vi "measure stable current.vi"(6 "measure transmission?":bool, 7 "na/V 2":dbl=1000.0, 8 "error in":errorcluster, 9 "measure ss":bool, 10 "field change wait(s)":u32=5, 11 "na/V":dbl=500.0) -> (0 "error out":errorcluster, 1 "stable current 2":dbl format="%.2f", 3 "stable current":dbl format="%.2f", 4 "inj current":dbl format="%#_6e", 5 "INJ ss ratio":dbl format="%#_6e")   [LabVIEW 2016]
uses:
  stable controls/stable cluster.ctl
  kubley/data acquisition 2009/beamline/controls/stable state combo.ctl
panel:
  in  "Start.Delay":dbl=2.0 format="%#_13g"
  in  "Charge State":dbl=3.0
  out "Waveform Graph 2":dbl[](graph)
  in  "stable data in":T1={"injector current"=1.0, "offset current"=1.0, "ss inj ratio"=1.0, "ss offset ratio"=1.0, "transmission"=1.0, "2nd offset current"=1.0}
  out "stable data out":T1={"injector current"=1.0, "offset current"=1.0, "ss inj ratio"=1.0, "ss offset ratio"=1.0, "transmission"=1.0, "2nd offset current"=1.0}
  out "stable current 3":cluster{"data":dbl[]}[](graph)
  in  "inj current 4":dbl
  out "inj current 3":dbl format="%#_6e"
  in  "inj current 2":dbl
  out "step":string
  in  "measure stable":bool
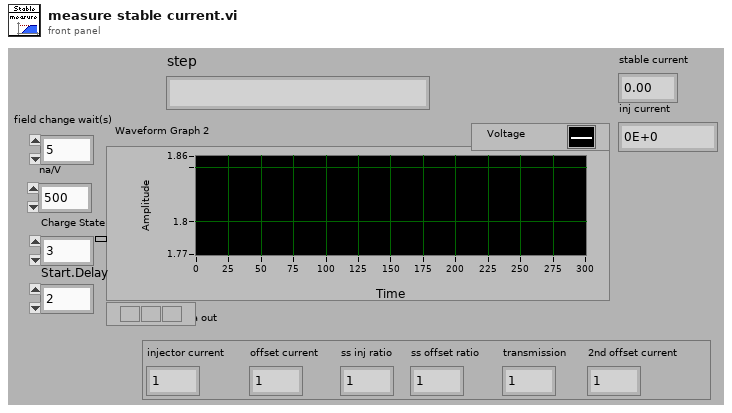
[diagram p1: front panel]
types:
  T1 = typedef "stable cluster.ctl" = cluster{"injector current":dbl, "offset current":dbl, "ss inj ratio":dbl, "ss offset ratio":dbl, "transmission":dbl, "2nd offset current":dbl}
  T2 = typedef "stable state combo.ctl" = string
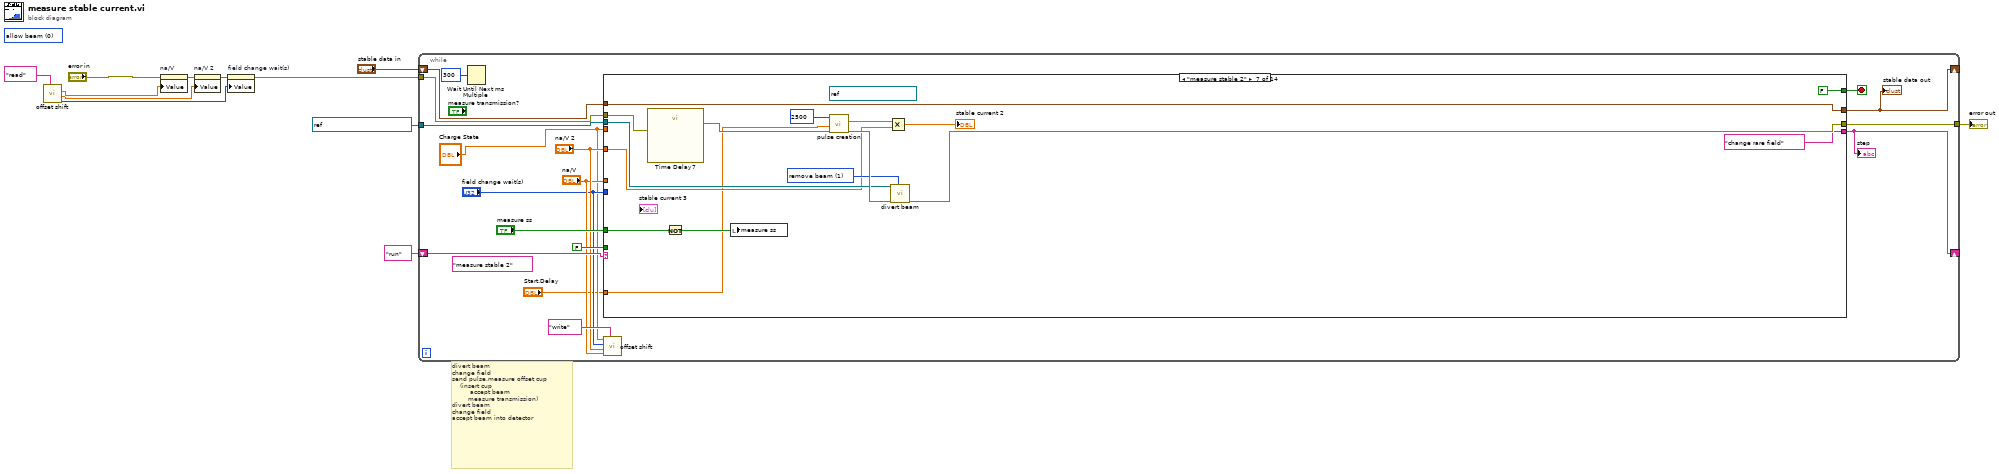
[diagram p0: block diagram]
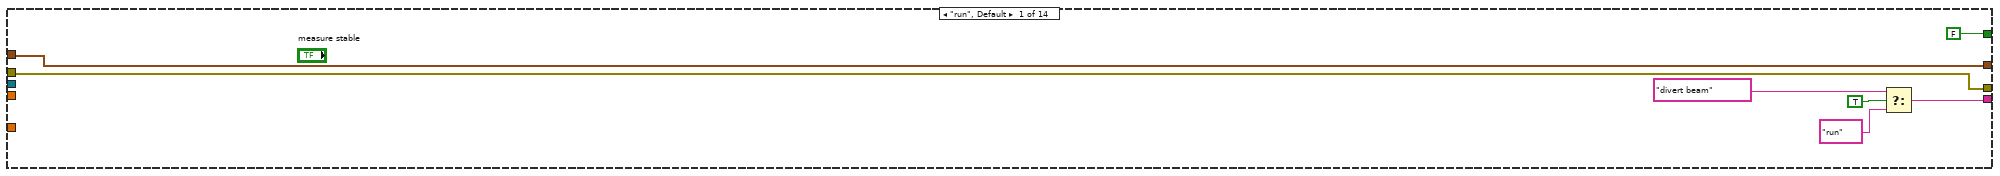
[diagram p2: hidden frame]
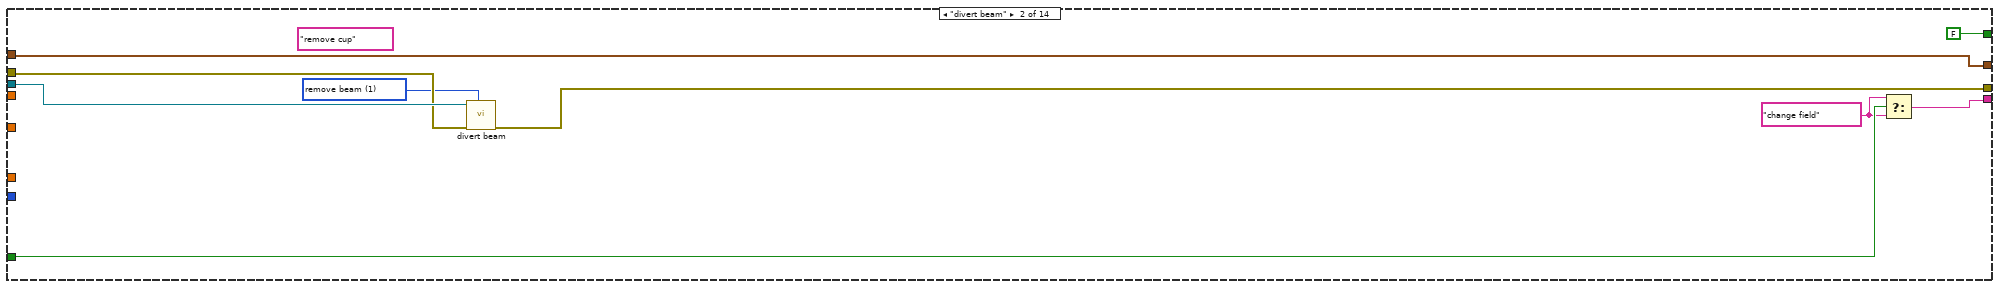
[diagram p3: hidden frame]
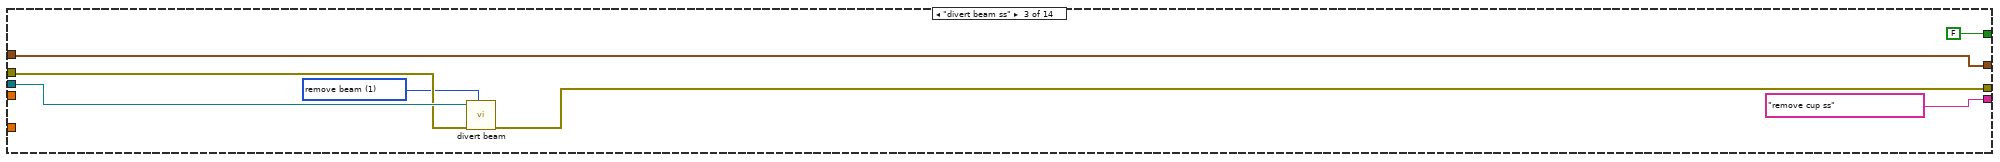
[diagram p4: hidden frame]
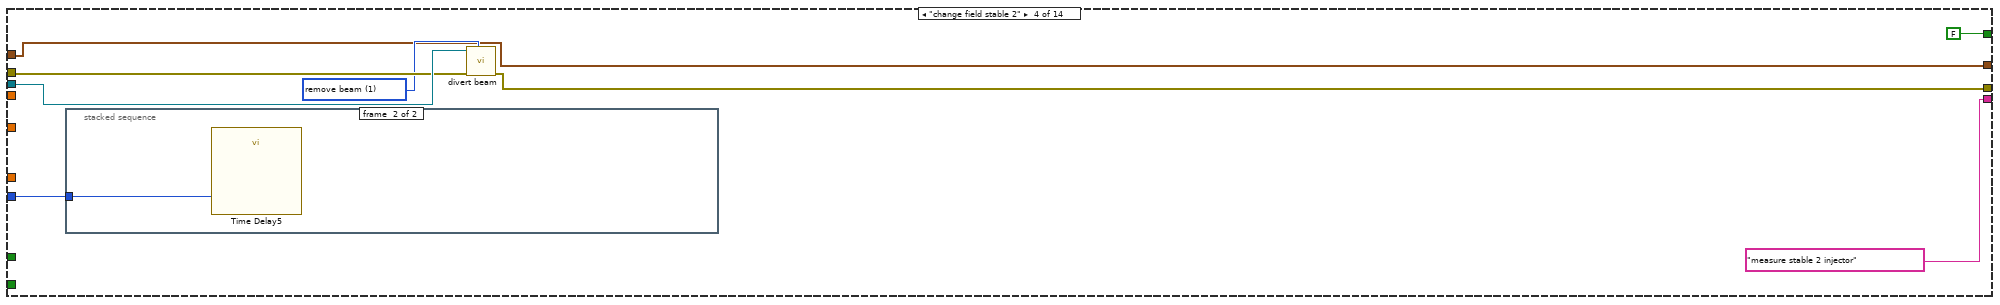
[diagram p5: hidden frame]
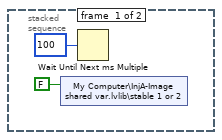
[diagram p6: hidden frame]
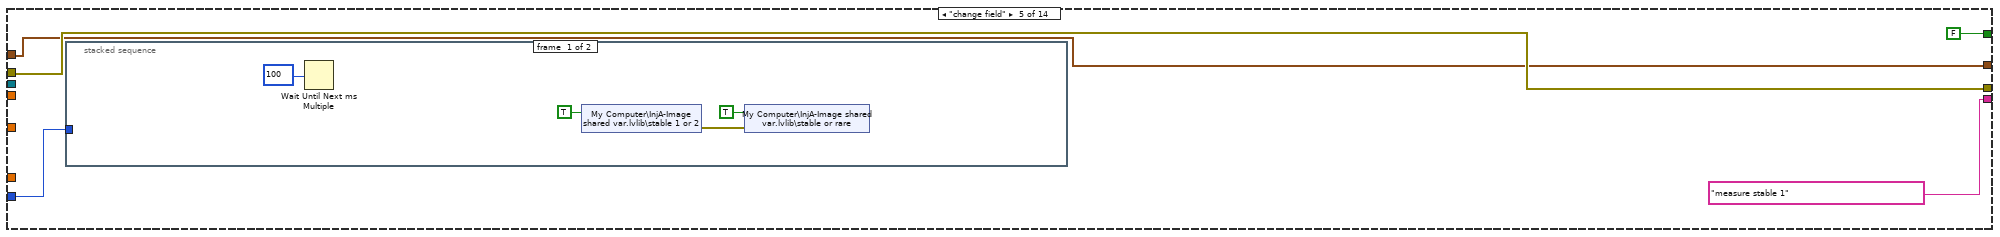
[diagram p7: hidden frame]
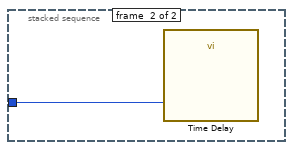
[diagram p8: hidden frame]
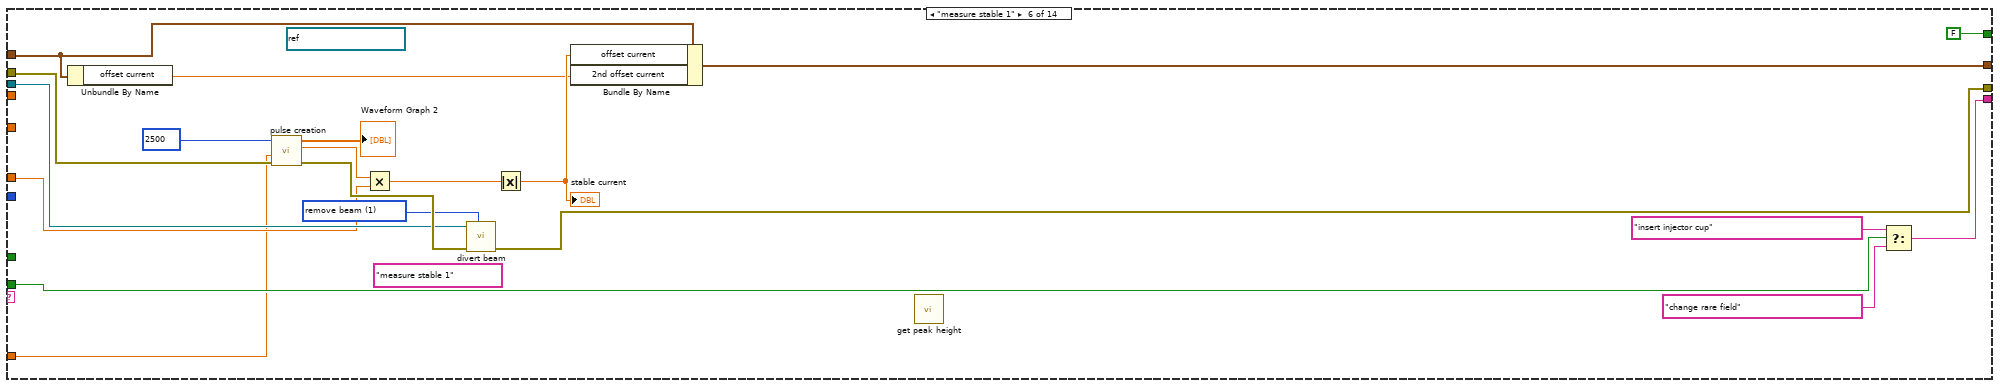
[diagram p9: hidden frame]
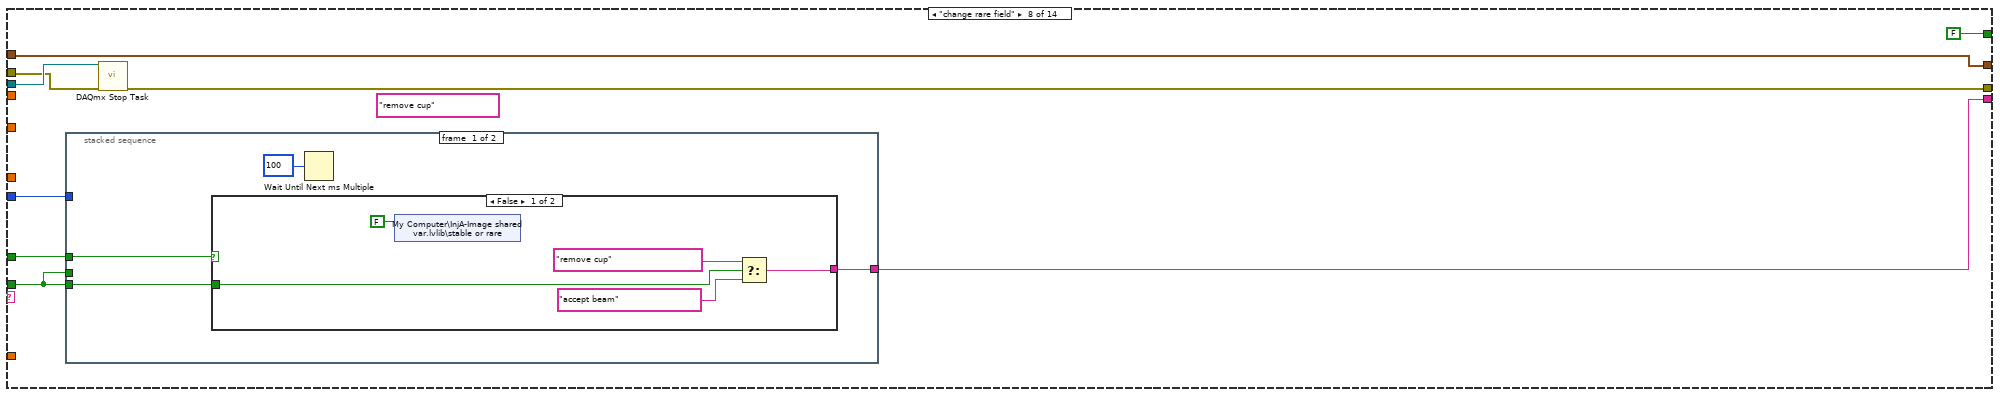
[diagram p10: hidden frame]
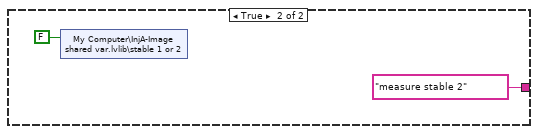
[diagram p11: hidden frame]
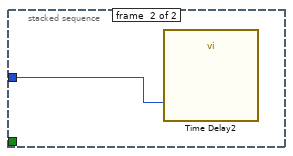
[diagram p12: hidden frame]
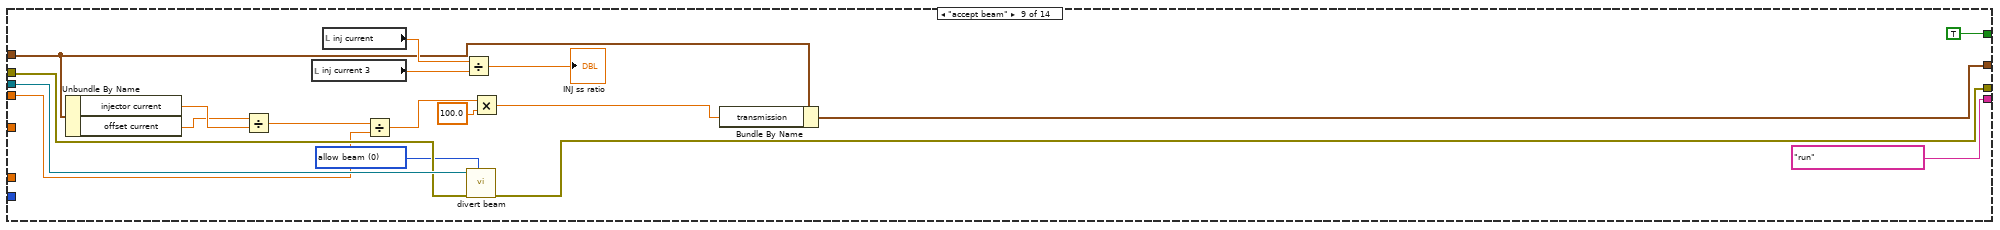
[diagram p13: hidden frame]
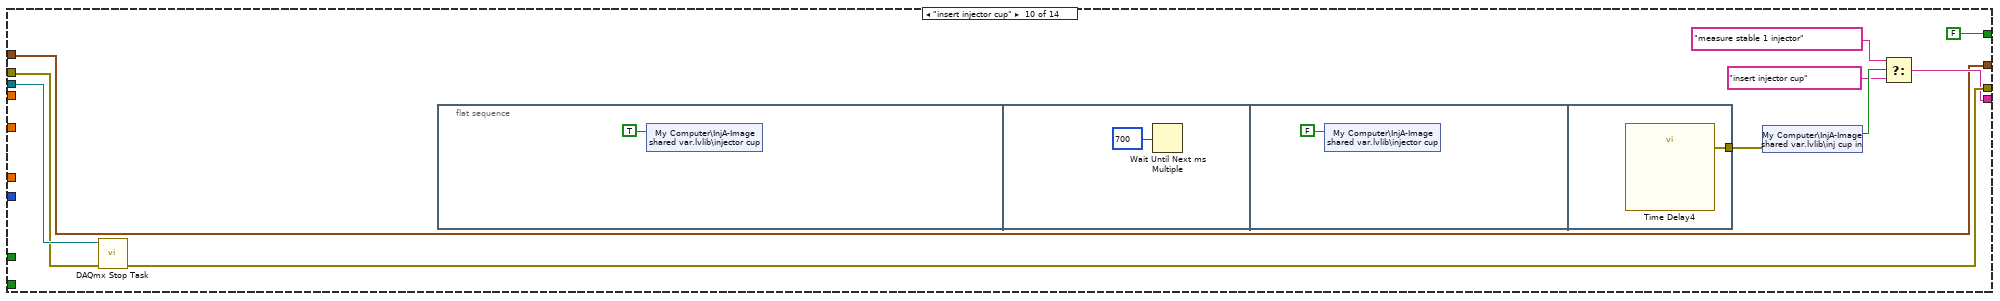
[diagram p14: hidden frame]
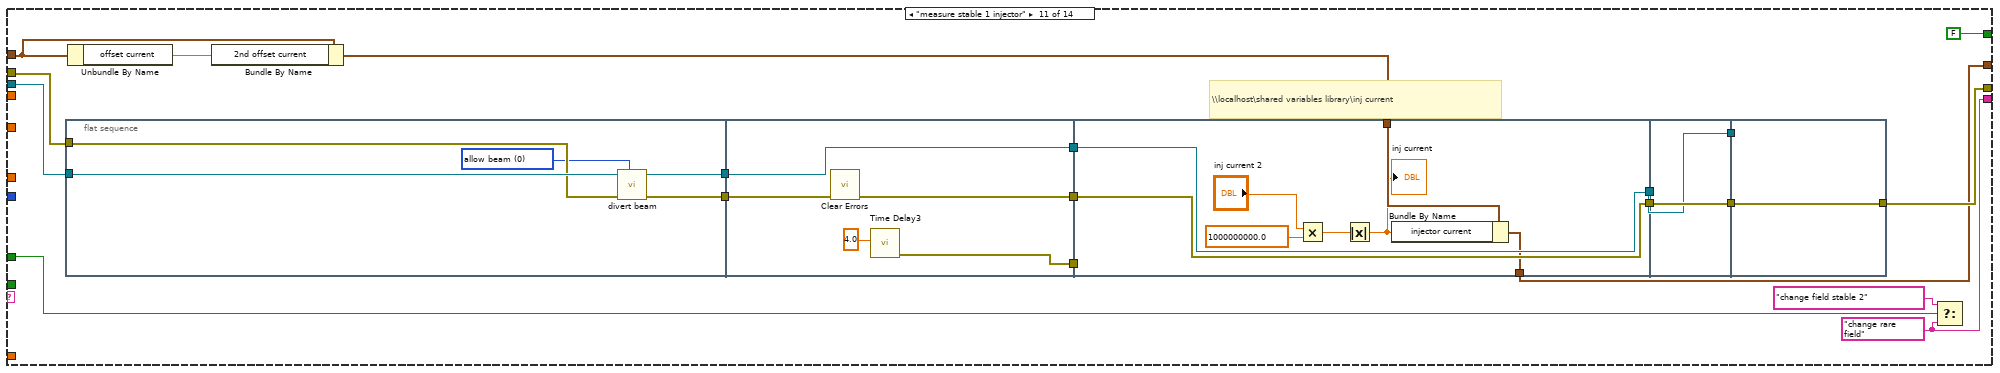
[diagram p15: hidden frame]
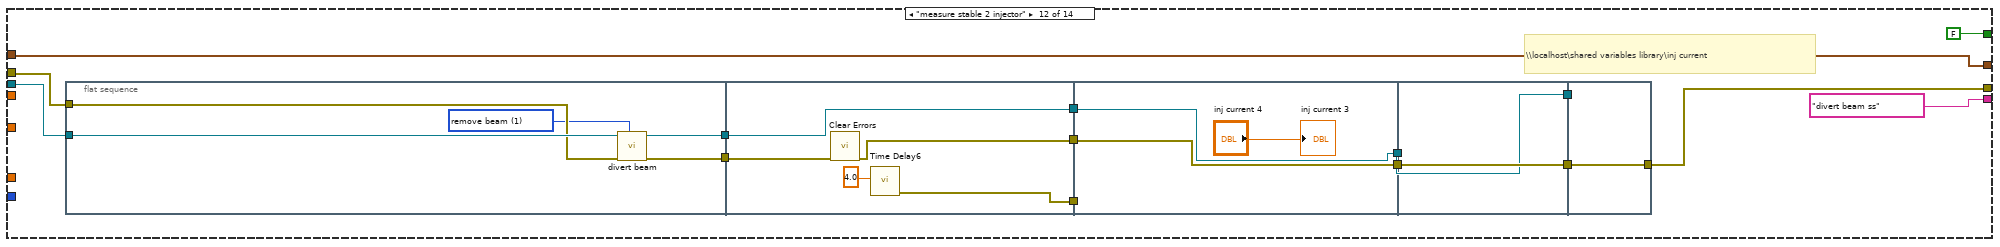
[diagram p16: hidden frame]
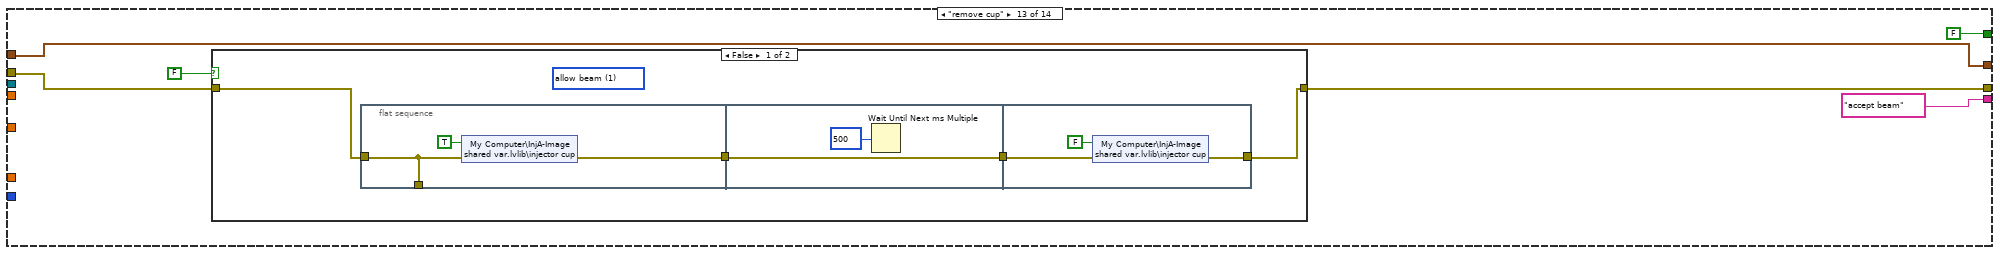
[diagram p17: hidden frame]
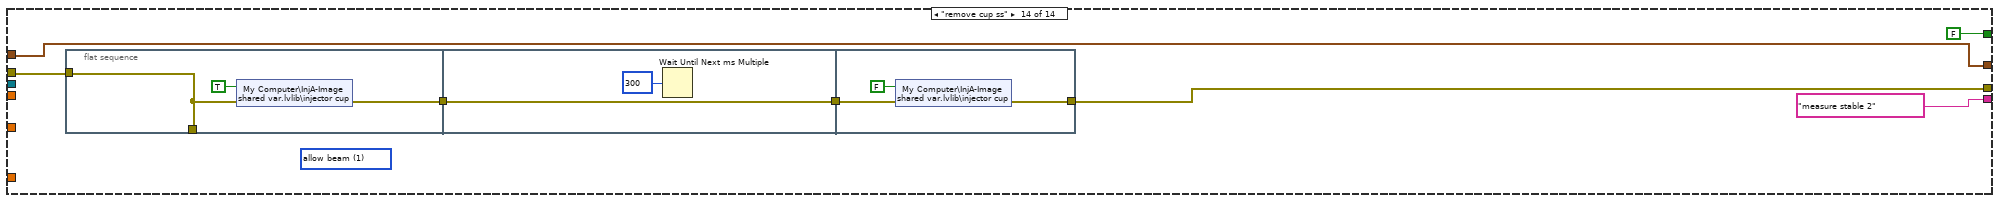
[diagram p19: hidden frame]
diagram:
  (unwired) u16 0 items=["allow beam", "remove beam"] ("divert beam? 2")
  # "divert beam\nchange field\nsend pulse,measure offset cup\n    (insert cup\n         accept beam\n        measure transmission)\ndivert beam\nchange field\naccept beam into detector"
  n1 = call "offset shift.vi"("read writ"="read") -> ("field change wait(s) out"=w5:u32, "na/V 2out"=w6:dbl, "na/V out"=w7:dbl)  [unwired: 7 in, 1 out]
  n2 = property on="na/V" class="DigNum (strict)"(error in="error in", "Value"=w7) -> (error out=w2:errorcluster)  [unwired: 1 in, 1 out]
  n3 = property on="na/V 2" class="DigNum (strict)"(error in=w2, "Value"=w6) -> (error out=w3:errorcluster)  [unwired: 1 in, 1 out]
  n4 = property on="field change wait(s)" class="DigNum (strict)"(error in=w3, "Value"=w5) -> (error out=w4:errorcluster)  [unwired: 1 in, 1 out]
  n5 = while {
    shift-right: [w28] -> _
    shift-left: T2 "run" ("stable measurement type") -> [w29]
    tunnel: refnum<k21> "stable current output" ("task/channels in") -> [w27]
    tunnel: [w25] -> w10
    tunnel: w4 -> [w24]
    shift-right: [w20] -> _
    shift-left: "stable data in" -> [w21]
    stop <- w23 stop-if-true
    (unwired) T2 "measure stable 2" ("stable measurement type")
    n6 = Wait Until Next ms Multiple(millisecond multiple=u32 300) -> ()  [unwired: 1 out]
    n7 = case shown="\"measure stable 2\"" w29 {
      tunnel: [w34 w40 T2 "remove cup ss" ("stable measurement type") T2 "measure stable 2 injector" ("stable measurement type") T2 "measure stable 1" ("stable measurement type") w84 T2 "change rare field" ("stable measurement type") w111 T2 "run" ("stable measurement type") w150 w167 T2 "divert beam ss" ("stable measurement type") T2 "accept beam" ("stable measurement type") T2 "measure stable 2" ("stable measurement type")] -> w28
      tunnel: w27 -> [_ w45 w52 w60 _ w89 w106 w116 w148 w157 w179 w215 _ _]
      tunnel: "field change wait(s)" -> [_ _ _ w55 w67 _ _ w118 _ _ _ _ _ _]
      tunnel: [FALSE ("stop") FALSE ("stop") FALSE ("stop") FALSE ("stop") FALSE ("stop") FALSE ("stop") FALSE ("stop") FALSE ("stop") TRUE ("stop") FALSE ("stop") FALSE ("stop") FALSE ("stop") FALSE ("stop") FALSE ("stop")] -> w23
      tunnel: [w31 w43 w50 w57 w65 w86 w104 w114 w144 w155 w170 w206 w237 w257] -> w25
      tunnel: w24 -> [w31 w42 w49 w56 w65 w90 w100 w115 w145 w156 w176 w212 w238 w258]
      tunnel: FALSE ("measure transmission?") -> [_ _ _ _ _ w88 _ w112 _ _ _ _ _ _]
      tunnel: "measure ss" -> [_ w41 _ _ _ _ w102 w113 _ _ w169 _ _ _]
      tunnel: w21 -> [w30 w37 w46 w53 w64 w78 w96 w110 w138 w149 w164 w204 w235 w254]
      tunnel: [w30 w37 w46 w53 w64 w79 w96 w110 w137 w149 w166 w204 w235 w254] -> w20
      tunnel: "Charge State" -> [_ _ _ _ _ _ _ _ w131 _ _ _ _ _]
      tunnel: "na/V" -> [_ _ _ _ _ w76 _ _ _ _ _ _ _ _]
      tunnel: "na/V 2" -> [_ _ _ _ _ _ w95 _ _ _ _ _ _ _]
      tunnel: "Start.Delay" -> [_ _ _ _ _ w74 w94 _ _ _ _ _ _ _]
      frame "run", Default {
        n8 = Select(t=T2 "divert beam" ("stable measurement type"), s=TRUE, f=T2 "run" ("stable measurement type")) -> (s? t:f=w34:T2)
      }
      frame "divert beam" {
        w38 = u16 1 items=["allow beam", "remove beam"] ("divert beam? 2")
        (unwired) T2 "remove cup" ("stable measurement type")
        w39 = T2 "change field" ("stable measurement type")
        n9 = call "divert beam.vi"("divert beam?"=w38, "error in"=w42, "task/channels in"=w45) -> ("error out"=w43:errorcluster)  [unwired: 7 in, 1 out]
        n10 = Select(t=w39, s=w41, f=w39) -> (s? t:f=w40:T2)
      }
      frame "divert beam ss" {
        w47 = u16 1 items=["allow beam", "remove beam"] ("divert beam? 2")
        n11 = call "divert beam.vi"("divert beam?"=w47, "error in"=w49, "task/channels in"=w52) -> ("error out"=w50:errorcluster)  [unwired: 7 in, 1 out]
      }
      frame "change field stable 2" {
        w54 = u16 1 items=["allow beam", "remove beam"] ("divert beam? 2")
        n12 = stacked-sequence {
          tunnel: w55 -> [_ w63]
          frame #0 {
            n13 = shared-variable "My Computer\\InjA-Image shared var.lvlib\\stable 1 or 2"(FALSE ("stable or rare")) -> ()  [unwired: 1 in, 1 out]
            n14 = Wait Until Next ms Multiple(millisecond multiple=u32 100) -> ()  [unwired: 1 out]
          }
          frame #1 {
            n15 = call "Time Delay5"("Delay Time (s)"=w63) -> ()  [unwired: 10 in, 1 out]
          }
        }
        n16 = call "divert beam.vi"("divert beam?"=w54, "error in"=w56, "task/channels in"=w60) -> ("error out"=w57:errorcluster)  [unwired: 7 in, 1 out]
      }
      frame "change field" {
        n17 = stacked-sequence {
          tunnel: w67 -> [_ w73]
          frame #0 {
            n18 = Wait Until Next ms Multiple(millisecond multiple=u32 100) -> ()  [unwired: 1 out]
            n19 = shared-variable "My Computer\\InjA-Image shared var.lvlib\\stable 1 or 2"(TRUE ("stable or rare")) -> (error out=w69:errorcluster)  [unwired: 1 in]
            n20 = shared-variable "My Computer\\InjA-Image shared var.lvlib\\stable or rare"(TRUE ("stable or rare"), error in=w69) -> ()  [unwired: 1 out]
          }
          frame #1 {
            n21 = call "Time Delay"("Delay Time (s)"=w73) -> ()  [unwired: 10 in, 1 out]
          }
        }
      }
      frame "measure stable 1" {
        w81 = u16 1 items=["allow beam", "remove beam"] ("divert beam? 2")
        (unwired) refnum<k21> "stable currents" ("task/channels in")
        (unwired) T2 "measure stable 1" ("stable measurement type")
        n22 = Unbundle By Name(w78) -> ("offset current"=w77:dbl)
        n23 = call "pulse creation.vi"("error in"=w90, "Start.Delay"=w74, "chopper width(usec)"=u32 2500) -> ("error out"=w92:errorcluster, "mean"=w82:dbl, "Waveform Graph 2"=→"Waveform Graph 2":dbl[])  [unwired: 4 in, 2 out]
        n24 = Multiply(x=w82, y=w76) -> (x*y=w83:dbl)
        n25 = call "divert beam.vi"("divert beam?"=w81, "error in"=w92, "task/channels in"=w89) -> ("error out"=w86:errorcluster)  [unwired: 7 in, 1 out]
        n26 = Absolute Value(x=w83) -> (abs(x)=w80:dbl)
        "stable current" <- w80
        n27 = Bundle By Name(cluster=w78, "offset current"=w80, "2nd offset current"=w77) -> (w79:T1)
        n28 = call "get peak height.vi"() -> ()  [unwired: 8 in, 4 out]
        n29 = Select(t=T2 "insert injector cup" ("stable measurement type"), s=w88, f=T2 "change rare field" ("stable measurement type")) -> (s? t:f=w84:T2)
      }
      frame "measure stable 2" {
        w97 = u16 1 items=["allow beam", "remove beam"] ("divert beam? 2")
        (unwired) refnum<k21> "secondary current" ("task/channels in")
        n30 = call "Time Delay7"("error in (no error)"=w100) -> ("error out"=w99:errorcluster)  [unwired: 10 in]
        n31 = Not(x=w102) -> (.not. x?=w101:bool)
        n32 = local write "measure ss"(w101) -> ()
        n33 = call "pulse creation.vi"("error in"=w99, "Start.Delay"=w94, "chopper width(usec)"=u32 2500) -> ("error out"=w108:errorcluster, "mean"=w98:dbl)  [unwired: 4 in, 3 out]
        n34 = Multiply(x=w98, y=w95) -> (x*y=→"stable current 2":dbl)
        n35 = call "divert beam.vi"("divert beam?"=w97, "error in"=w108, "task/channels in"=w106) -> ("error out"=w104:errorcluster)  [unwired: 7 in, 1 out]
      }
      frame "change rare field" {
        (unwired) T2 "remove cup" ("stable measurement type")
        n36 = stacked-sequence {
          tunnel: w118 -> [_ w130]
          tunnel: w113 -> [w121 _]
          tunnel: w112 -> [w120 _]
          tunnel: w112 -> [_ _]
          tunnel: [w119 _] -> w111
          frame #0 {
            n37 = case shown="False" w121 {
              tunnel: w120 -> [w124 _]
              tunnel: [w123 T2 "measure stable 2" ("stable measurement type")] -> w119
              frame False {
                n38 = shared-variable "My Computer\\InjA-Image shared var.lvlib\\stable or rare"(FALSE ("stable or rare")) -> ()  [unwired: 1 in, 1 out]
                n39 = Select(t=T2 "remove cup" ("stable measurement type"), s=w124, f=T2 "accept beam" ("stable measurement type")) -> (s? t:f=w123:T2)
              }
              frame True {
                n40 = shared-variable "My Computer\\InjA-Image shared var.lvlib\\stable 1 or 2"(FALSE ("stable or rare")) -> ()  [unwired: 1 in, 1 out]
              }
            }
            n41 = Wait Until Next ms Multiple(millisecond multiple=u32 100) -> ()  [unwired: 1 out]
          }
          frame #1 {
            n42 = call "Time Delay2"("Delay Time (s)"=w130) -> ()  [unwired: 10 in, 1 out]
          }
        }
        n43 = call <vilib>:"DAQmx Stop Task.vi"("task/channels in"=w116, "error in"=w115) -> ("error out"=w114:errorcluster)  [unwired: 12 in, 1 out]
      }
      frame "accept beam" {
        w140 = u16 0 items=["allow beam", "remove beam"] ("divert beam? 2")
        n44 = Unbundle By Name(w138) -> ("injector current"=w136:dbl, "offset current"=w135:dbl)
        n45 = Divide(x=w135, y=w136) -> (x/y=w139:dbl)
        n46 = local read "inj current 3"() -> (w142:dbl)
        n47 = local read "inj current"() -> (w143:dbl)
        n48 = Divide(x=w139, y=w131) -> (x/y=w134:dbl)
        n49 = Divide(x=w143, y=w142) -> (x/y=→"INJ ss ratio":dbl)
        n50 = call "divert beam.vi"("divert beam?"=w140, "error in"=w145, "task/channels in"=w148) -> ("error out"=w144:errorcluster)  [unwired: 7 in, 1 out]
        n51 = Multiply(x=w134, y=100.0) -> (x*y=w132:dbl)
        n52 = Bundle By Name(cluster=w138, "transmission"=w132) -> (w137:T1)
      }
      frame "insert injector cup" {
        n53 = call <vilib>:"DAQmx Stop Task.vi"("task/channels in"=w157, "error in"=w156) -> ("error out"=w155:errorcluster)  [unwired: 12 in, 1 out]
        n54 = flat-sequence {
          tunnel: [w162] -> w154
          frame #0 {
            n55 = shared-variable "My Computer\\InjA-Image shared var.lvlib\\injector cup"(TRUE ("injector cup")) -> ()  [unwired: 1 in, 1 out]
          }
          frame #1 {
            n56 = Wait Until Next ms Multiple(millisecond multiple=u32 700) -> ()  [unwired: 1 out]
          }
          frame #2 {
            n57 = shared-variable "My Computer\\InjA-Image shared var.lvlib\\injector cup"(FALSE ("injector cup")) -> ()  [unwired: 1 in, 1 out]
          }
          frame #3 {
            n58 = call "Time Delay4"() -> ("error out"=w162:errorcluster)  [unwired: 11 in]
          }
        }
        n59 = shared-variable "My Computer\\InjA-Image shared var.lvlib\\inj cup in"(error in=w154) -> (w153:bool)  [unwired: 1 out]
        n60 = Select(t=T2 "measure stable 1 injector" ("stable measurement type"), s=w153, f=T2 "insert injector cup") -> (s? t:f=w150:T2)
      }
      frame "measure stable 1 injector" {
        w167 = T2 "change rare field" ("stable measurement type")
        # "\\\\localhost\\shared variables library\\inj current"
        n61 = flat-sequence {
          tunnel: w179 -> [w187]
          tunnel: [w186] -> w180
          tunnel: [w184] -> w177
          tunnel: w176 -> [w185]
          tunnel: [w190] -> w181
          tunnel: w180 -> [w191]
          tunnel: [w192] -> w178
          tunnel: w177 -> [w192]
          tunnel: [w188] -> w171
          tunnel: [w200] -> w175
          tunnel: w181 -> [w200]
          tunnel: [w199] -> w173
          tunnel: w178 -> [w199]
          tunnel: w171 -> [_]
          tunnel: w163 -> [w198]
          tunnel: [w197] -> w166
          tunnel: w175 -> [w202]
          tunnel: [w202] -> w174
          tunnel: w173 -> [w201]
          tunnel: [w201] -> w172
          tunnel: w174 -> [w203]
          tunnel: w172 -> [_]
          tunnel: [w203] -> w170
          frame #0 {
            w183 = u16 0 items=["allow beam", "remove beam"] ("divert beam? 2")
            n62 = call "divert beam.vi"("divert beam?"=w183, "error in"=w185, "task/channels in"=w187) -> ("error out"=w186:errorcluster, "task out"=w184:refnum<k21>)  [unwired: 7 in]
          }
          frame #1 {
            n63 = call <vilib>:"Clear Errors.vi"("error in (no error)"=w191) -> ("error out"=w190:errorcluster)  [unwired: 5 in, 1 out]
            n64 = call "Time Delay3"("Delay Time (s)"=4.0) -> ("error out"=w188:errorcluster)  [unwired: 10 in]
          }
          frame #2 {
            n65 = Multiply(x="inj current 2", y=1000000000.0) -> (x*y=w194:dbl)
            n66 = Absolute Value(x=w194) -> (abs(x)=w193:dbl)
            "inj current" <- w193
            n67 = Bundle By Name(cluster=w198, "injector current"=w193) -> (w197:T1)
          }
          frame #3 {
          }
          frame #4 {
          }
        }
        n68 = Unbundle By Name(w164) -> ("offset current"=w165:dbl)
        n69 = Bundle By Name(cluster=w164, "2nd offset current"=w165) -> (w163:T1)
        n70 = Select(t=T2 "change field stable 2" ("stable measurement type"), s=w169, f=w167) -> ()  [unwired: 1 out]
      }
      frame "measure stable 2 injector" {
        # "\\\\localhost\\shared variables library\\inj current"
        n71 = flat-sequence {
          tunnel: w215 -> [w223]
          tunnel: [w222] -> w216
          tunnel: [w220] -> w213
          tunnel: w212 -> [w221]
          tunnel: [w226] -> w217
          tunnel: w216 -> [w227]
          tunnel: [w228] -> w214
          tunnel: w213 -> [w228]
          tunnel: [w224] -> w207
          tunnel: [w231] -> w211
          tunnel: w217 -> [w231]
          tunnel: [w230] -> w209
          tunnel: w214 -> [w230]
          tunnel: w207 -> [_]
          tunnel: w211 -> [w233]
          tunnel: [w233] -> w210
          tunnel: w209 -> [w232]
          tunnel: [w232] -> w208
          tunnel: w210 -> [w234]
          tunnel: w208 -> [_]
          tunnel: [w234] -> w206
          frame #0 {
            w219 = u16 1 items=["allow beam", "remove beam"] ("divert beam? 2")
            n72 = call "divert beam.vi"("divert beam?"=w219, "error in"=w221, "task/channels in"=w223) -> ("error out"=w222:errorcluster, "task out"=w220:refnum<k21>)  [unwired: 7 in]
          }
          frame #1 {
            n73 = call <vilib>:"Clear Errors.vi"("error in (no error)"=w227) -> ("error out"=w226:errorcluster)  [unwired: 5 in, 1 out]
            n74 = call "Time Delay6"("Delay Time (s)"=4.0) -> ("error out"=w224:errorcluster)  [unwired: 10 in]
          }
          frame #2 {
            "inj current 3" <- "inj current 4"
          }
          frame #3 {
          }
          frame #4 {
          }
        }
      }
      frame "remove cup" {
        n75 = case shown="False" FALSE {
          tunnel: w238 -> [w242 w253]
          tunnel: [w241 w253] -> w237
          frame False {
            (unwired) u16 1 items=["divert beam", "allow beam"] ("divert beam? 2")
            n76 = flat-sequence {
              tunnel: [w245] -> _
              tunnel: w242 -> [w245]
              tunnel: [w246] -> w244
              tunnel: [w248] -> w243
              tunnel: w244 -> [w248]
              tunnel: w243 -> [w251]
              tunnel: [w250] -> w241
              frame #0 {
                n77 = shared-variable "My Computer\\InjA-Image shared var.lvlib\\injector cup"(TRUE ("injector cup"), error in=w245) -> (error out=w246:errorcluster)
              }
              frame #1 {
                n78 = Wait Until Next ms Multiple(millisecond multiple=u32 500) -> ()  [unwired: 1 out]
              }
              frame #2 {
                n79 = shared-variable "My Computer\\InjA-Image shared var.lvlib\\injector cup"(FALSE ("injector cup"), error in=w251) -> (error out=w250:errorcluster)
              }
            }
          }
          frame True {
          }
        }
      }
      frame "remove cup ss" {
        (unwired) u16 1 items=["divert beam", "allow beam"] ("divert beam? 2")
        n80 = flat-sequence {
          tunnel: [w261] -> _
          tunnel: w258 -> [w261]
          tunnel: [w262] -> w256
          tunnel: [w264] -> w255
          tunnel: w256 -> [w264]
          tunnel: w255 -> [w267]
          tunnel: [w266] -> w257
          frame #0 {
            n81 = shared-variable "My Computer\\InjA-Image shared var.lvlib\\injector cup"(TRUE ("injector cup"), error in=w261) -> (error out=w262:errorcluster)
          }
          frame #1 {
            n82 = Wait Until Next ms Multiple(millisecond multiple=u32 300) -> ()  [unwired: 1 out]
          }
          frame #2 {
            n83 = shared-variable "My Computer\\InjA-Image shared var.lvlib\\injector cup"(FALSE ("injector cup"), error in=w267) -> (error out=w266:errorcluster)
          }
        }
      }
    }
    "step" <- w28
    "stable data out" <- w20
    n84 = call "offset shift.vi"("read writ"="write", "na/V"="na/V", "na/V 2"="na/V 2", "field change wait(s)"="field change wait(s)", "charge state"="Charge State") -> ()  [unwired: 3 in, 4 out]
  }
  "error out" <- w10
